vi "EPS-Request Data.vi"(4 "Access Mode":T1, 6 "Timeout":i32=2000, 8 "error in":errorcluster, 10 "Requst Data":string, 11 "EPS Setting In":T2) -> (0 "error out":errorcluster, 2 "Response Data":string, 3 "EPS Setting Out":T2)   [LabVIEW 2018]
uses:
  Data Def/EPS-Setting.ctl
  Data Def/EPS-Access Mode.ctl
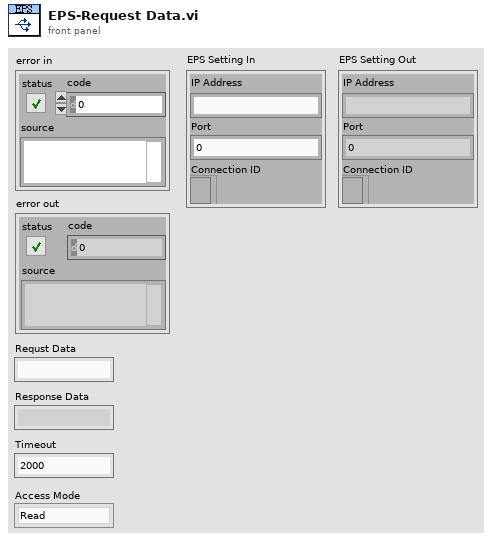
[diagram p1: front panel]
types:
  T1 = typedef "EPS-Access Mode.ctl" = enum16{"Read", "Write"}
  T2 = typedef "EPS-Setting.ctl" = cluster{"IP Address":string, "Port":u16, "Connection ID":refnum<k5>}
  T3 = enum16{"Standard", "Buffered", "CRLF", "Immediate"}
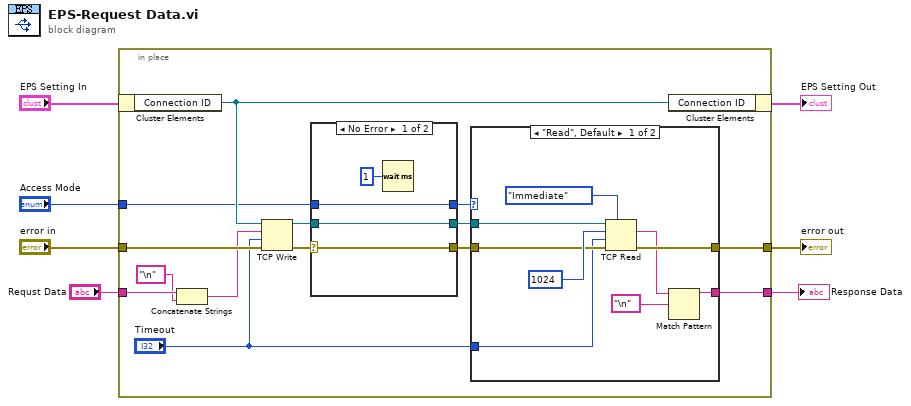
[diagram p0: block diagram]
diagram:
  n1 = in-place {
    in-place-border: "error in" -> [w20]
    in-place-border: "Requst Data" -> [w16]
    in-place-border: [w18] -> w3
    in-place-border: [w17] -> w2
    in-place-border: "Access Mode" -> [w9]
    n2 = in-place-cluster #1("EPS Setting In") -> ("Connection ID"=w21:refnum<k5>)
    n3 = Concatenate Strings(w16, "\n" ("string")) -> (w14:string)
    n4 = TCP Write(connection ID=w21, data in=w14, error in (no error)=w20, 9:"Timeout") -> (connection ID out=w11:refnum<k5>, error out=w13:errorcluster)  [unwired: 1 out]
    n5 = case shown="No Error" w13 {
      selector: w13 -> [w25 w28]
      tunnel: [w25 w28] -> w12
      tunnel: w11 -> [w24 w27]
      tunnel: [w24 w27] -> w10
      tunnel: w9 -> [w23 w26]
      tunnel: [w23 w26] -> w8
      frame No Error {
        n6 = Wait (ms)(milliseconds to wait=u32 1) -> ()  [unwired: 1 out]
      }
      frame Error {
      }
    }
    n7 = case shown="\"Read\", Default" w8 {
      tunnel: w12 -> [w36 w38]
      tunnel: w10 -> [w35 _]
      tunnel: "Timeout" -> [w33 _]
      tunnel: [w32 w38] -> w18
      tunnel: [w29 _] -> w17
      frame "Read", Default {
        n8 = TCP Read(connection ID=w35, bytes to read=1024 ("Bytes zu lesen"), error in (no error)=w36, 7:T3."Immediate" ("Modus (Standard)"), 9:w33) -> (data out=w31:string, error out=w32:errorcluster)  [unwired: 1 out]
        n9 = Match Pattern(string=w31, regular expression="\n" ("string")) -> (before substring=w29:string)  [unwired: 1 in, 3 out]
      }
      frame "Write" {
      }
    }
    n10 = in-place-cluster #1("Connection ID"=w21) -> (→"EPS Setting Out":T2)
  }
  "error out" <- w3
  "Response Data" <- w2
